vi "PBI_MFA_Interface_DriveBusVolts1.vi"() -> (3 "DriveBusVolts_0V":sgl)   [LabVIEW 2018]
panel:
  out "error DriveBusVolts_0V":errorcluster
  out "AAABuild":i32
  in  "MintController":refnum<k7>(container)
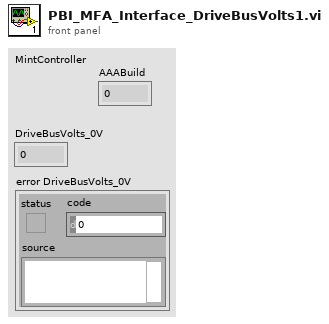
[diagram p1: front panel]
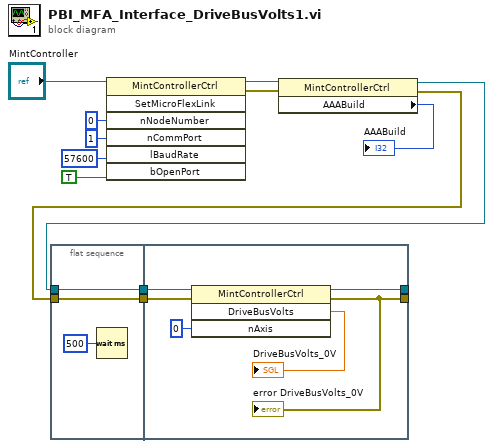
[diagram p0: block diagram]
diagram:
  n1 = flat-sequence {
    tunnel: [w15] -> w3
    tunnel: [w14] -> w2
    tunnel: w4 -> [w15]
    tunnel: w1 -> [w14]
    tunnel: [w17] -> _
    tunnel: w3 -> [w21]
    tunnel: w2 -> [w18]
    tunnel: [w16] -> _
    frame #0 {
      n2 = Wait (ms)(milliseconds to wait=u32 500) -> ()  [unwired: 1 out]
    }
    frame #1 {
      n3 = invoke class="MintControllerCtrl" method="DriveBusVolts"(reference=w21, error in=w18, "nAxis"=i16 0) -> (reference out=w16:refnum<k7>, error out=w17:errorcluster, "DriveBusVolts"=→"DriveBusVolts_0V":sgl)  [unwired: 1 in, 1 out]
      "error DriveBusVolts_0V" <- w17
    }
  }
  n4 = invoke class="MintControllerCtrl" method="SetMicroFlexLink"(reference="MintController", "nNodeNumber"=i16 0, "nCommPort"=i16 1, "lBaudRate"=57600, "bOpenPort"=TRUE) -> (reference out=w12:refnum<k7>, error out=w6:errorcluster)  [unwired: 2 in, 5 out]
  n5 = property class="MintControllerCtrl"(reference=w12, error in=w6) -> (reference out=w4:refnum<k7>, error out=w1:errorcluster, "AAABuild"=→"AAABuild":i32)
